vi "FromString.vi"(8 "error in (no error)":errorcluster, 11 "ResultProcessor Config in":refnum<class "ResultProcessor Config.lvclass">) -> (0 "error out":errorcluster, 3 "ResultProcessor Config out":refnum<class "ResultProcessor Config.lvclass">)   [LabVIEW 2015, in "ResultProcessor Config.lvclass"]
uses:
  ResultProcessor Config.lvclass
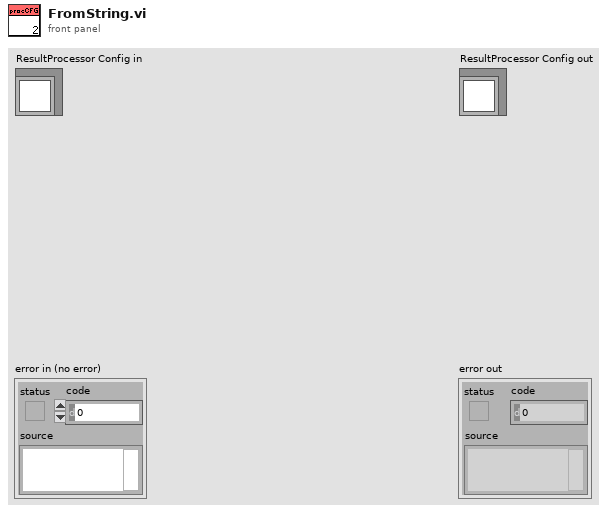
[diagram p1: front panel]
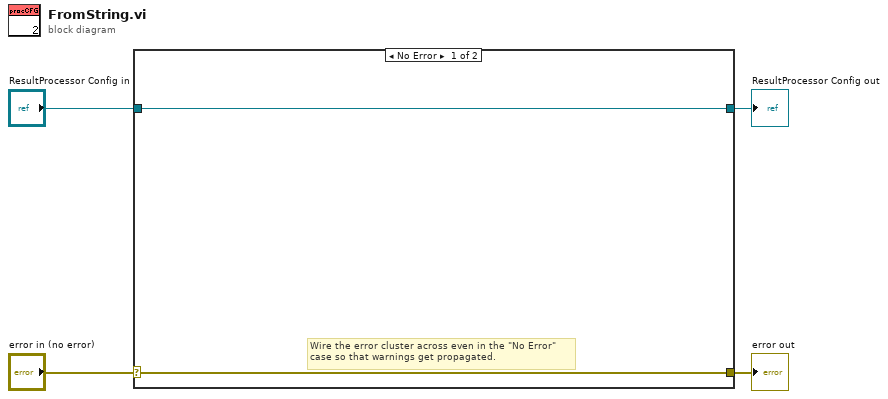
[diagram p0: block diagram]
diagram:
  n1 = case shown="No Error" "error in (no error)" {
    selector: "error in (no error)" -> [w5 w8]
    tunnel: [w5 w8] -> w3
    tunnel: [w6 w7] -> w1
    tunnel: "ResultProcessor Config in" -> [w6 w7]
    frame No Error {
      # "Wire the error cluster across even in the \"No Error\"\ncase so that warnings get propagated."
    }
    frame Error {
    }
  }
  "error out" <- w3
  "ResultProcessor Config out" <- w1
